vi "OMA_Query.vi"(0 "System no.":i32=1 min=1 max=4 step=1, 2 "Axes to query":string[](array[string]), 3 "All axes?":bool, 4 "Axis identifier?":bool=TRUE, 5 "error in":errorcluster) -> (14 "Target position":dbl[](array[numeric]) format="%.6f", 19 "error out":errorcluster)   [LabVIEW 2020]
doc: "Returns commanded open-loop target position.\n\nE-861: If All axes? = TRUE, then Axis identifier? can be FALSE\n\nE-871, E-873: If All axes? = TRUE, then Axis identifier? can be FALSE."
panel:
  # "Returns commanded open-loop target position."
  # "If all axes: use"
  # "Query"
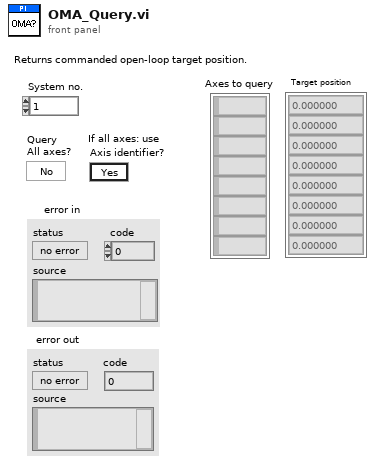
[diagram p1: front panel]
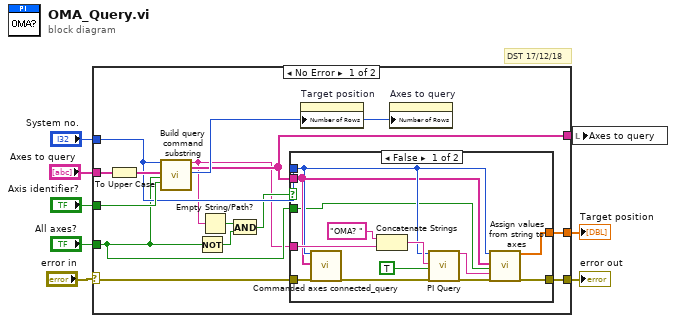
[diagram p0: block diagram]
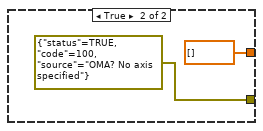
[diagram p2: hidden frame]
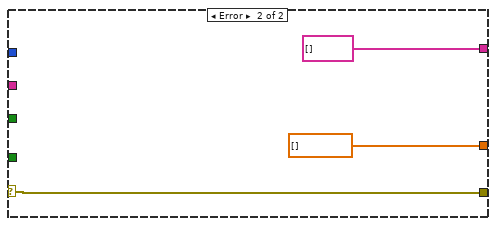
[diagram p3: hidden frame]
diagram:
  # "DST 17/12/18"
  n1 = case shown="No Error" "error in" {
    selector: "error in" -> [w9 w38]
    tunnel: [w22 dbl[] [] ("Values")] -> w8
    tunnel: "Axes to query" -> [w21 _]
    tunnel: [w20 w38] -> w6
    tunnel: "Axis identifier?" -> [w18 _]
    tunnel: "System no." -> [w16 _]
    tunnel: [w15 string[] [] ("Axes to query out")] -> w3
    tunnel: "All axes?" -> [w14 _]
    frame No Error {
      n2 = To Upper Case(1:w21) -> (0:w19:string[])
      n3 = call "Build query command substring.vi"("System no."=w16, "Axes to query in"=w19, "Query\nAll axes?"=w14, "For all axes: use\nAxis identifier?"=w18) -> ("Command substring"=w11:string, "Axes to query out"=w15:string[], "Number of rows"=w17:u32)  [unwired: 2 in, 11 out]
      n4 = Not(x=w14) -> (.not. x?=w13:bool)
      n5 = Empty String/Path?(string/path=w11) -> (empty?=w10:bool)
      n6 = And(x=w10, y=w13) -> (x .and. y?=w12:bool)
      n7 = case shown="False" w12 {
        tunnel: [w32 dbl[] [] ("Values")] -> w22
        tunnel: w9 -> [w31 _]
        tunnel: [w26 errorcluster {"status"=TRUE, "code"=100, "source"="OMA? No axis specified"} ("error out")] -> w20
        tunnel: w11 -> [w30 _]
        tunnel: w16 -> [w29 _]
        tunnel: w15 -> [w28 _]
        tunnel: w14 -> [w27 _]
        frame False {
          n8 = call "Commanded axes connected_query.vi"("System no."=w29, "Commanded axes"=w28, "error in"=w31) -> ("error out"=w25:errorcluster)  [unwired: 1 in, 15 out]
          n9 = Concatenate Strings("OMA? ", w30) -> (w33:string)
          n10 = call "PI Query.vi"("System no."=w29, "String to send"=w33, "Attach termination char.?"=TRUE ("Attach Linefeed?"), "error in"=w25) -> ("String read"=w24:string, "error out"=w23:errorcluster)  [unwired: 3 in, 11 out]
          n11 = call "Assign values from string to axes.vi"("System no."=w29, "Queried axes"=w28, "All axes queried?"=w27, "Input String"=w24, "error in"=w23) -> ("Values"=w32:dbl[], "error out"=w26:errorcluster)  [unwired: 4 in, 9 out]
        }
        frame True {
        }
      }
      n12 = property on="Target position" class="Arr (strict)"("Number of Rows"=w17) -> ()  [unwired: 2 in, 2 out]
      n13 = property on="Axes to query" class="Arr (strict)"("Number of Rows"=w17) -> ()  [unwired: 2 in, 2 out]
    }
    frame Error {
    }
  }
  "error out" <- w6
  "Target position" <- w8
  n14 = local write "Axes to query"(w3) -> ()
